vi "1motorPwmTest.vi"() -> ()   [LabVIEW 2019]
uses:
  builds/KNRm_ReMi_Toolkit/KNRm/KNRm_ReMi_OS6/home/lvuser/natinst/bin/KNRm_ReMi_OS6.lvlibp/KNRm_ReMi_Toolkit/Control/MotorNumberSelect.ctl
  builds/KNRm_ReMi_Toolkit/KNRm/KNRm_ReMi_OS6/home/lvuser/natinst/bin/KNRm_ReMi_OS6.lvlibp
panel:
  out "flash":bool
  out "Time has Elapsed":bool
  out "ENC (deg)":dbl
  in  "Horizontal Pointer Slide":dbl(slide) scale=-100.0..100.0
  in  "Reset":bool
  in  "Stop Button":bool
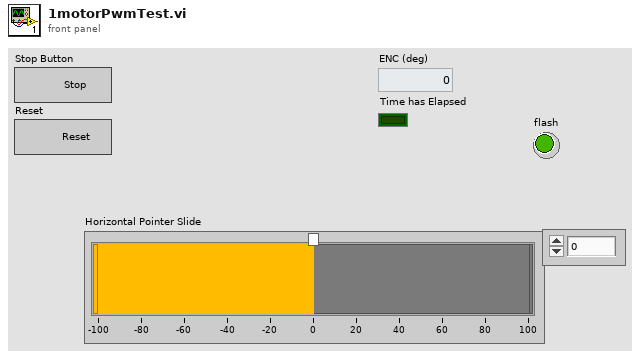
[diagram p1: front panel]
types:
  T1 = cluster{"Numeric":u8, "Numeric":u8, "Numeric":u8, "Numeric":u8}
  T2 = typedef "KNRm_ReMi_OS6.lvlibp/MotorNumberSelect.ctl" = enum16{"DS1", "DS2", "DS3", "DS4"}
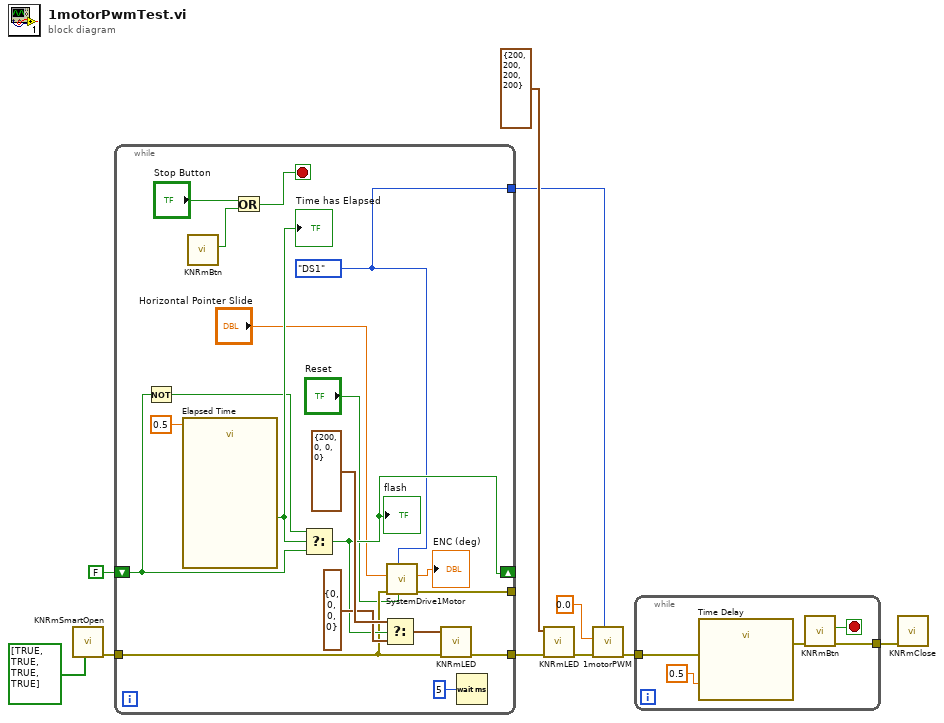
[diagram p0: block diagram]
diagram:
  n1 = call "KNRmSmartOpen.vi"("DS1-4 Mode (T: Speed/ F: PWM)"=bool[] [TRUE, TRUE, TRUE, TRUE] ("SpeedMode")) -> ("error out"=w10:errorcluster)  [unwired: 7 in, 3 out]
  n2 = while {
    tunnel: w10 -> [w16]
    tunnel: [w15] -> _
    shift-right: [w19] -> _
    shift-left: FALSE -> [w23]
    tunnel: [w17] -> w7
    tunnel: [w13] -> w4
    stop <- w26 stop-if-true
    w13 = MotorNumberSelect."DS1" ("MotorNumberSelect")
    n3 = Not(x=w23) -> (.not. x?=w22:bool)
    n4 = call "Elapsed Time"("Time Target (s)"=0.5) -> ("Time has Elapsed"=w24:bool)  [unwired: 11 in, 7 out]
    "Time has Elapsed" <- w24
    n5 = call "KNRmBtn.vi"() -> ("KNRm(myRIO)Button"=w27:bool)  [unwired: 10 in, 1 out]
    n6 = Or(x="Stop Button", y=w27) -> (x .or. y?=w26:bool)
    n7 = Select(t=w22, s=w24, f=w23) -> (s? t:f=w19:bool)
    "flash" <- w19
    n8 = Select(t=T1 {"Numeric"=200, "Numeric"=0, "Numeric"=0, "Numeric"=0} ("LEDSet"), s=w19, f=T1 {"Numeric"=0, "Numeric"=0, "Numeric"=0, "Numeric"=0} ("LEDSet")) -> (s? t:f=w18:T1)
    n9 = call "SystemDrive1Motor.vi"("Reset"="Reset", "MotorNumberSelect"=w13, "error in"=w16, "Motor(deg/s)"="Horizontal Pointer Slide") -> ("error out"=w15:errorcluster, "ENC (deg)"=→"ENC (deg)":dbl)  [unwired: 6 in]
    n10 = call "KNRmLED.vi"("error in"=w16, "LEDSet"=w18) -> ("error out"=w17:errorcluster)  [unwired: 9 in]
    n11 = Wait (ms)(milliseconds to wait=u32 5) -> ()  [unwired: 1 out]
  }
  n12 = call "KNRmLED.vi"("error in"=w7, "LEDSet"=T1 {"Numeric"=200, "Numeric"=200, "Numeric"=200, "Numeric"=200}) -> ("error out"=w3:errorcluster)  [unwired: 9 in]
  n13 = call "1motorPWM.vi"("MotorNumberSelect"=w4, "error in"=w3, "MotorSpeed(PWM%)"=0.0) -> ("error out"=w2:errorcluster)  [unwired: 7 in, 1 out]
  n14 = while {
    tunnel: w2 -> [w32]
    tunnel: [w33] -> w1
    stop <- w34 stop-if-true
    n15 = call "Time Delay"("error in (no error)"=w32, "Delay Time (s)"=0.5) -> ("error out"=w31:errorcluster)  [unwired: 9 in]
    n16 = call "KNRmBtn.vi"("error in"=w31) -> ("error out"=w33:errorcluster, "KNRm(myRIO)Button"=w34:bool)  [unwired: 9 in]
  }
  n17 = call "KNRmClose.vi"("error in"=w1) -> ()  [unwired: 10 in, 1 out]
